vi "Write_TTTR_header.vi"(0 "TTTR Ref In":refnum<file>, 1 "TXTHDR":T11, 2 "BINHDR_P":T3, 3 "BINHDR_H":T7, 4 "BOARDHDR":T4, 5 "Error In":errorcluster, 6 "TTTRHDR_P":T6, 7 "MAINHARDWAREHDR":T8, 8 "TTTRHDR_H":T10, 9 "ICSETINGS":T9, 10 "IMGHDR":T1, 12 "LSMHDR":T2) -> (14 "TTTR Ref Out":refnum<file>, 19 "Error Out":errorcluster)   [LabVIEW 2012]
uses:
  Online correlation/TTTR_data_headers/TXTHDR.ctl
  Online correlation/TTTR_data_headers/BINHDR_H.ctl
  Online correlation/TTTR_data_headers/MAINHARDWAREHDR.ctl
  Online correlation/TTTR_data_headers/ICSETTINGS.ctl
  Online correlation/TTTR_data_headers/TTTRHDR_H.ctl
  Online correlation/TTTR_data_headers/IMGHDR.ctl
  Online correlation/TTTR_data_headers/LSMHDR.ctl
  Online correlation/TTTR_data_headers/BINHDR_P.ctl
  Online correlation/TTTR_data_headers/BOARDHDR.ctl
  Online correlation/TTTR_data_headers/RtChan.ctl
  Online correlation/TTTR_data_headers/TTTRHDR_P.ctl
panel:
  out "Scan Type":enum32{"IMG", "LSM"}(tab)
  out "Data Type":enum32{"PicoHarp 300", "HydraHarp 400"}(tab)
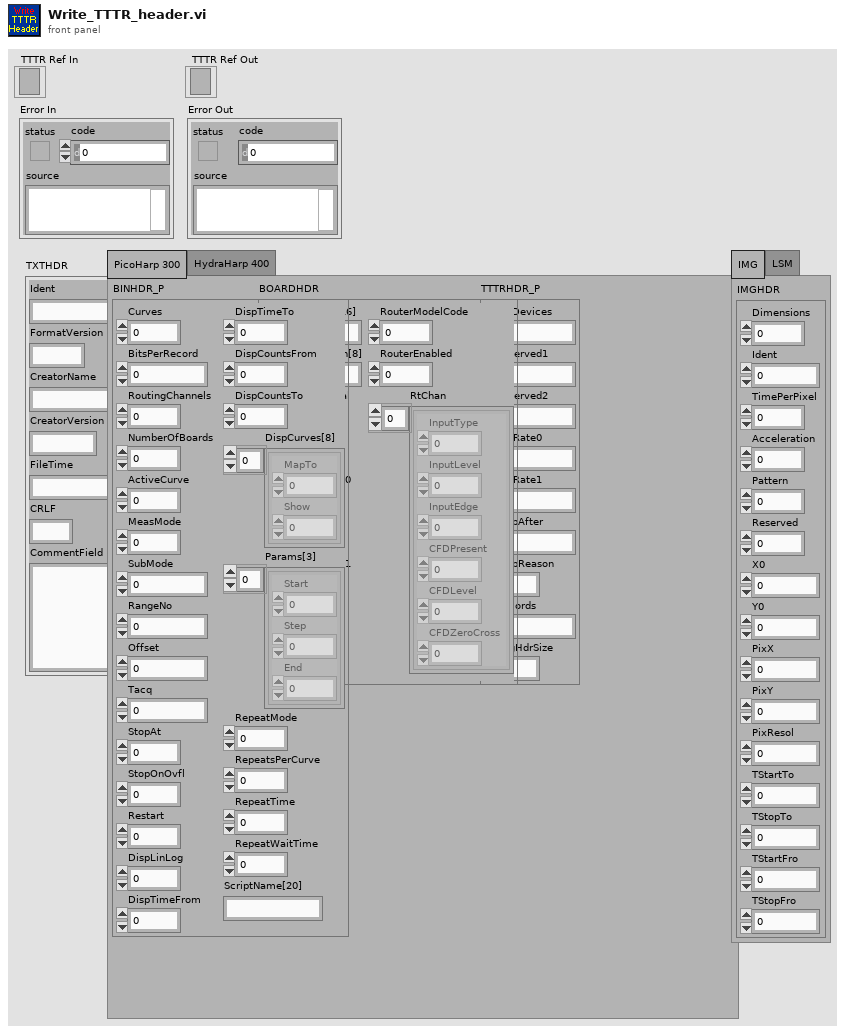
[diagram p1: front panel]
types:
  T1 = typedef "IMGHDR.ctl" = cluster{"Dimensions":i32, "Ident":i32, "TimePerPixel":i32, "Acceleration":i32, "Pattern":i32, "Reserved":i32, "X0":sgl, "Y0":sgl, "PixX":i32, "PixY":i32, "PixResol":sgl, "TStartTo":sgl, "TStopTo":sgl, "TStartFro":sgl, "TStopFro":sgl}
  T2 = typedef "LSMHDR.ctl" = cluster{"Dimensions":i32, "Ident":i32, "Frame":i32, "LineStart":i32, "LineStop":i32, "Pattern":u8, "prcSin":u8, "prcStart":u8, "prcStop":u8, "PixX":i32, "PixY":i32, "Resolution":sgl}
  T3 = typedef "BINHDR_P.ctl" = cluster{"Curves":i32, "BitsPerRecord":i32, "RoutingChannels":i32, "NumberOfBoards":i32, "ActiveCurve":i32, "MeasMode":i32, "SubMode":i32, "RangeNo":i32, "Offset":i32, "Tacq":i32, "StopAt":i32, "StopOnOvfl":i32, "Restart":i32, "DispLinLog":i32, "DispTimeFrom":i32, "DispTimeTo":i32, "DispCountsFrom":i32, "DispCountsTo":i32, "DispCurves[8]":cluster{"MapTo":i32, "Show":i32}[], "Params[3]":cluster{"Start":sgl, "Step":sgl, "End":sgl}[], "RepeatMode":i32, "RepeatsPerCurve":i32, "RepeatTime":i32, "RepeatWaitTime":i32, "ScriptName[20]":string}
  T4 = typedef "BOARDHDR.ctl" = cluster{"HardwareIdent[16]":string, "HardwareVersion[8]":string, "HardwareSerial":i32, "SyncDivider":i32, "CFDZeroCross0":i32, "CFDLevel0":i32, "CFDZeroCross1":i32, "CFDLevel1":i32, "Resolution":sgl, "RouterModelCode":i32, "RouterEnabled":i32, "RtChan":T5}
  T5 = typedef "RtChan.ctl" = cluster{"InputType":i32, "InputLevel":i32, "InputEdge":i32, "CFDPresent":i32, "CFDLevel":i32, "CFDZeroCross":i32}[]
  T6 = typedef "TTTRHDR_P.ctl" = cluster{"ExtDevices":i32, "Reserved1":i32, "Reserved2":i32, "CntRate0":i32, "CntRate1":i32, "StopAfter":i32, "StopReason":i32, "Records":u32, "ImgHdrSize":i32}
  T7 = typedef "BINHDR_H.ctl" = cluster{"Curves":i32, "BitsPerRecord":i32, "ActiveCurve":i32, "MeasMode":i32, "SubMode":i32, "Binning":i32, "Resolution":dbl, "Offset":i32, "Tacq":i32, "StopAt":i32, "StopOnOvfl":i32, "Restart":i32, "DispLinLog":i32, "DispTimeFrom":i32, "DispTimeTo":i32, "DispCountsFrom":i32, "DispCountsTo":i32, "DispCurves[8]":cluster{"MapTo":i32, "Show":i32}[], "Params[3]":cluster{"Start":sgl, "Step":sgl, "End":sgl}[], "RepeatMode":i32, "RepeatsPerCurve":i32, "RepeatTime":i32, "RepeatWaitTime":i32, "ScriptName[20]":string}
  T8 = typedef "MAINHARDWAREHDR.ctl" = cluster{"HardwareIdent[16]":string, "HardwarePartNo[8]":string, "HardwareSerial":i32, "nModulesPresent":i32, "ModuleInfo[10]":cluster{"MapTo":i32, "Show":i32}[], "BaseResolution":dbl, "InputsEnabled":u64, "InpChansPresent":i32, "RefClockSource":i32, "ExtDevices":i32, "MarkerSettings":i32, "SyncDivider":i32, "SyncCFDLevel":i32, "SyncCFDZeroCross":i32, "SyncOffset":i32}
  T9 = typedef "ICSETTINGS.ctl" = cluster{"ICSETTINGS":cluster{"InputModuleIndex":i32, "InputCFDLevel":i32, "InputCFDZeroCross":i32, "InputOffset":i32}[], "InputRate":i32[]}
  T10 = typedef "TTTRHDR_H.ctl" = cluster{"SyncRate":i32, "StopAfter":i32, "StopReason":i32, "ImgHdrSize":i32, "nRecords":u64}
  T11 = typedef "TXTHDR.ctl" = cluster{"Ident":string, "FormatVersion":string, "CreatorName":string, "CreatorVersion":string, "FileTime":string, "CRLF":string, "CommentField":string}
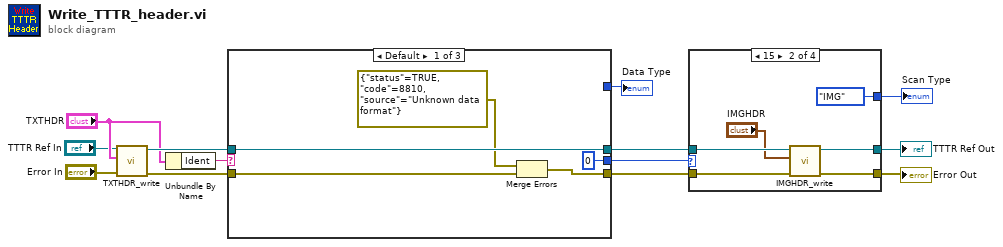
[diagram p0: block diagram]
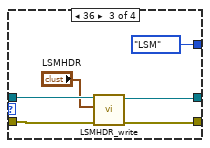
[diagram p3: hidden frame]
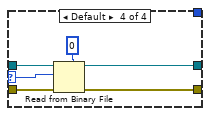
[diagram p4: hidden frame]
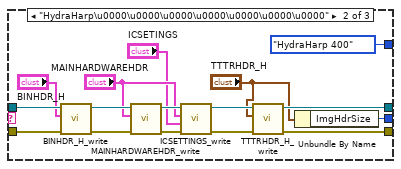
[diagram p5: hidden frame]
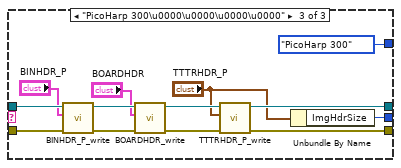
[diagram p6: hidden frame]
diagram:
  n1 = call "TXTHDR_write.vi"("error in (no error)"="Error In", "TXTHDR"="TXTHDR", "refnum in"="TTTR Ref In") -> ("error out"=w13:errorcluster, "refnum out"=w12:refnum<file>)  [unwired: 7 in]
  n2 = Unbundle By Name("TXTHDR") -> ("Ident"=w8:string)
  n3 = case shown="Default" w8 {
    tunnel: w13 -> [w17 w34 w47]
    tunnel: w12 -> [w18 w33 w46]
    tunnel: [w15 w25 w40] -> w11
    tunnel: [w18 w24 w41] -> w10
    tunnel: [0 ("ImgHdrSize") w22 w38] -> w7
    tunnel: [_ enum32{"PicoHarp 300", "HydraHarp 400"}."HydraHarp 400" ("Data Type") enum32{"PicoHarp 300", "HydraHarp 400"}."PicoHarp 300" ("Data Type")] -> w1
    frame Default {
      n4 = Merge Errors(errorcluster {"status"=TRUE, "code"=8810, "source"="Unknown data format"} ("error out"), w17) -> (w15:errorcluster)
    }
    frame "HydraHarp\u0000\u0000\u0000\u0000\u0000\u0000\u0000" {
      n5 = call "BINHDR_H_write.vi"("error in (no error)"=w34, "BINHDR_H"="BINHDR_H", "refnum in"=w33) -> ("error out"=w32:errorcluster, "refnum out"=w31:refnum<file>)  [unwired: 7 in]
      n6 = call "MAINHARDWAREHDR_write.vi"("error in (no error)"=w32, "MAINHARDWAREHDR"="MAINHARDWAREHDR", "refnum in"=w31) -> ("error out"=w30:errorcluster, "refnum out"=w29:refnum<file>)  [unwired: 7 in]
      n7 = call "ICSETTINGS_write.vi"("error in (no error)"=w30, "ICSETINGS"="ICSETINGS", "MAINHARDWAREHDR"="MAINHARDWAREHDR", "refnum in"=w29) -> ("error out"=w27:errorcluster, "refnum out"=w26:refnum<file>)  [unwired: 6 in]
      n8 = call "TTTRHDR_H_write.vi"("error in (no error)"=w27, "TTTRHDR_H"="TTTRHDR_H", "refnum in"=w26) -> ("error out"=w25:errorcluster, "refnum out"=w24:refnum<file>)  [unwired: 7 in]
      n9 = Unbundle By Name("TTTRHDR_H") -> ("ImgHdrSize"=w22:i32)
    }
    frame "PicoHarp 300\u0000\u0000\u0000\u0000" {
      n10 = call "BINHDR_P_write.vi"("error in (no error)"=w47, "BINHDR_P"="BINHDR_P", "refnum in"=w46) -> ("error out"=w45:errorcluster, "refnum out"=w44:refnum<file>)  [unwired: 7 in]
      n11 = call "BOARDHDR_write.vi"("error in (no error)"=w45, "BOARDHDR"="BOARDHDR", "refnum in"=w44) -> ("error out"=w43:errorcluster, "refnum out"=w42:refnum<file>)  [unwired: 7 in]
      n12 = call "TTTRHDR_P_write.vi"("error in (no error)"=w43, "TTTRHDR_P"="TTTRHDR_P", "refnum in"=w42) -> ("error out"=w40:errorcluster, "refnum out"=w41:refnum<file>)  [unwired: 7 in]
      n13 = Unbundle By Name("TTTRHDR_P") -> ("ImgHdrSize"=w38:i32)
    }
  }
  "Data Type" <- w1
  n14 = case shown="15" w7 {
    selector: w7 -> [_ _ _ w63]
    tunnel: w11 -> [w49 w55 w61 w67]
    tunnel: [w49 w54 w58 w66] -> w3
    tunnel: w10 -> [w48 w53 w60 w65]
    tunnel: [w48 w52 w59 w64] -> w4
    tunnel: [_ enum32{"IMG", "LSM"}."IMG" ("Scan Type") enum32{"IMG", "LSM"}."LSM" ("Scan Type") _] -> w2
    frame 0 {
    }
    frame 15 {
      n15 = call "IMGHDR_write.vi"("error in (no error)"=w55, "IMGHDR"="IMGHDR", "refnum in"=w53) -> ("error out"=w54:errorcluster, "refnum out"=w52:refnum<file>)  [unwired: 7 in]
    }
    frame 36 {
      n16 = call "LSMHDR_write.vi"("error in (no error)"=w61, "LSMHDR"="LSMHDR", "refnum in"=w60) -> ("error out"=w58:errorcluster, "refnum out"=w59:refnum<file>)  [unwired: 7 in]
    }
    frame Default {
      n17 = Read from Binary File(5:0 ("ImgHdrSize"), 8:w67, 10:w63, 11:w65) -> (0:w66:errorcluster, 3:w64:refnum<file>)  [unwired: 2 in, 2 out]
    }
  }
  "TTTR Ref Out" <- w4
  "Error Out" <- w3
  "Scan Type" <- w2
